vi "Test Get Named Range Values (String).vi"(11 "Test Case In":refnum<class "Test Open Xml.lvclass">) -> (0 "error out":errorcluster, 3 "Test Case Out":refnum<class "Test Open Xml.lvclass">)   [LabVIEW 2025, in "Test Open Xml.lvclass"]
uses:
  Test Open Xml.lvclass
  C:/Program Files/National Instruments/LabVIEW 2025/vi.lib/Astemes/LUnit/Test Case.lvclass
  <vilib>/Astemes/LUnit/Test Case.lvclass/Test Case.ctl
  e7d09ce7-04db-40ce-9c4e-a78b31ec9fe8.vi
  <vilib>/Astemes/LUnit/Append Pass Result.vi
  <vilib>/Astemes/LUnit/Append Fail Result.vi
  e7d09ce7-04db-40ce-9c4e-a78b31ec9fe8.vi/9c5d11cd-9439-4240-a1ee-d9baace9c924.vi
  <vilib>/Astemes/LUnit/Run In UI.vi
  <vilib>/Utility/error.llb/Clear Errors.vi
  Test Open Xml.lvclass/Test Open Xml.ctl
  Source/Open Xml.lvlib
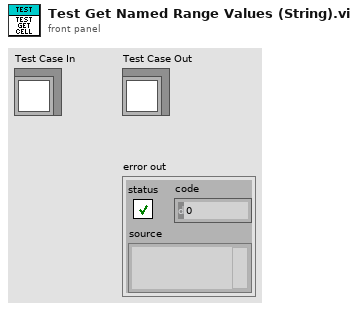
[diagram p1: front panel]
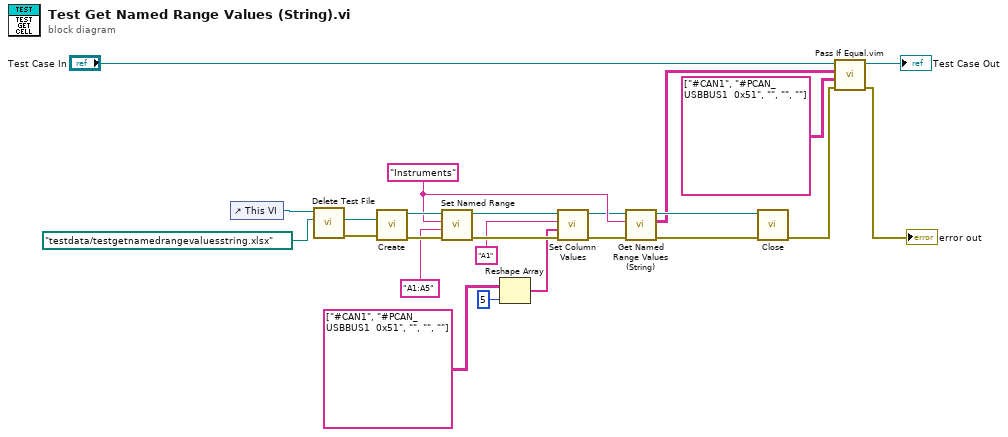
[diagram p0: block diagram]
diagram:
  w9 = "Instruments" ("Range Identifier")
  n1 = control-ref of="This VI"() -> (w12:refnum<vi>)
  n2 = call "Delete Test File.vi"("name or relative path"=path "testdata/testgetnamedrangevaluesstring.xlsx", "VI in"=w12) -> ("error out"=w15:errorcluster, "deleted path"=w14:path)  [unwired: 8 in]
  n3 = call "Create.vi"("error in"=w15, "Path"=w14) -> ("error out"=w21:errorcluster, "SpreadsheetDoc"=w10:refnum<k24>)  [unwired: 8 in]
  n4 = call "Set Named Range.vi"("error in"=w21, "Cell Range"="A1:A5", "Named Range Identifier"=w9, "SpreadsheetDoc in"=w10) -> ("error out"=w11:errorcluster, "SpreadsheetDoc out"=w6:refnum<k24>)  [unwired: 6 in]
  n5 = Reshape Array(string[][] [["#CAN1"], ["#PCAN_USBBUS1  0x51"], [""], [""], [""]] ("Cells"), 5 ("dimension size")) -> (w1:string[])
  n6 = call "Set Column Values.vi"("error in"=w11, "Values"=w1, "Cell Address"="A1", "SpreadsheetDoc"=w6) -> ("error out"=w7:errorcluster, "SpreadsheetDoc out"=w5:refnum<k24>)  [unwired: 6 in]
  n7 = call "Get Named Range Values (String).vi"("error in"=w7, "Named Range Identifier"=w9, "SpreadsheetDocument"=w5) -> ("error out"=w20:errorcluster, "Cells"=w17:string[][], "SpreadsheetDocument out"=w18:refnum<k24>)  [unwired: 6 in]
  n8 = call "Close.vi"("error in"=w20, "SpreadsheetDoc"=w18) -> ("error out"=w19:errorcluster)  [unwired: 9 in]
  n9 = call "Pass If Equal.vim"("error in (no error)"=w19, "Actual"=string[][] [["#CAN1"], ["#PCAN_USBBUS1  0x51"], [""], [""], [""]] ("Cells"), "Expected"=w17, "LUnit Test Case In"="Test Case In") -> ("error out"=→"error out":errorcluster, "LUnit Test Case Out"=→"Test Case Out":refnum<class "Test Open Xml.lvclass">)  [unwired: 6 in]
